vi "wd_repalceInIndex (DBL).vi"(6 "data type":T7, 7 "data":dbl[](array[numeric]), 8 "error in (no error)":errorcluster, 9 "value index":u64, 10 "channel index":u32, 11 "meta in":T1={"TargetFile"=path "", "StreamMode"=enum."File", "Append?"=FALSE, "ChunkSize"=0, "TimeColumnMode"=enum."Empty", "TimestampFormat"="", "AbsoluteTime?"=FALSE, "FileAttribute "={"Creator"="", "Title"="", "SheetName"=""}, "Column"=[], "FileRef"=refnum, "MemoryRef"=[], "RecordInfo"=[], " ChannelPreviousInfo"=[], "ChannelFirstRecord"=[], "PredefinedFormattedValueLength"=20, "DiskTemplate"={"XMLRef"=[refnum, refnum, refnum, refnum, refnum, refnum], "ZipPath"=path "", "MetaFile"={"Ref"=refnum, "NextRow"=0, "NextPosition"=0, "Block"=[]}, "TempFolder"=path ""}}) -> (0 "error out":errorcluster, 3 "meta out":T1={"TargetFile"=path "", "StreamMode"=enum."File", "Append?"=FALSE, "ChunkSize"=0, "TimeColumnMode"=enum."Empty", "TimestampFormat"="", "AbsoluteTime?"=FALSE, "FileAttribute "={"Creator"="", "Title"="", "SheetName"=""}, "Column"=[], "FileRef"=refnum, "MemoryRef"=[], "RecordInfo"=[], " ChannelPreviousInfo"=[], "ChannelFirstRecord"=[], "PredefinedFormattedValueLength"=20, "DiskTemplate"={"XMLRef"=[refnum, refnum, refnum, refnum, refnum, refnum], "ZipPath"=path "", "MetaFile"={"Ref"=refnum, "NextRow"=0, "NextPosition"=0, "Block"=[]}, "TempFolder"=path ""}})   [LabVIEW 2020, in "NI_ExcelFile.lvlib"]
uses:
  <vilib>/express/express shared/NI_ExcelFile/NI_ExcelFile.lvlib
  <vilib>/express/express shared/NI_ExcelFile/Ctrls/DataType.ctl
  <vilib>/express/express shared/NI_ExcelFile/Ctrls/MainData.ctl
  <vilib>/express/express shared/NI_ExcelFile/Ctrls/StreamMode.ctl
  <vilib>/express/express shared/NI_ExcelFile/Ctrls/TimeColumnMode.ctl
  <vilib>/express/express shared/NI_ExcelFile/Ctrls/FileAttribute.ctl
  <vilib>/express/express shared/NI_ExcelFile/Ctrls/Columns.ctl
  <vilib>/express/express shared/NI_ExcelFile/Ctrls/ColumnInfo.ctl
  <vilib>/express/express shared/NI_ExcelFile/Ctrls/wd_recordInfo.ctl
  <vilib>/express/express shared/NI_ExcelFile/Ctrls/disk_TemplateFile.ctl
  <vilib>/express/express shared/NI_ExcelFile/Ctrls/meta_file.ctl
  <vilib>/express/express shared/NI_ExcelFile/Ctrls/meta_Block.ctl
  <vilib>/express/express shared/NI_ExcelFile/Ctrls/meta_BlockType.ctl
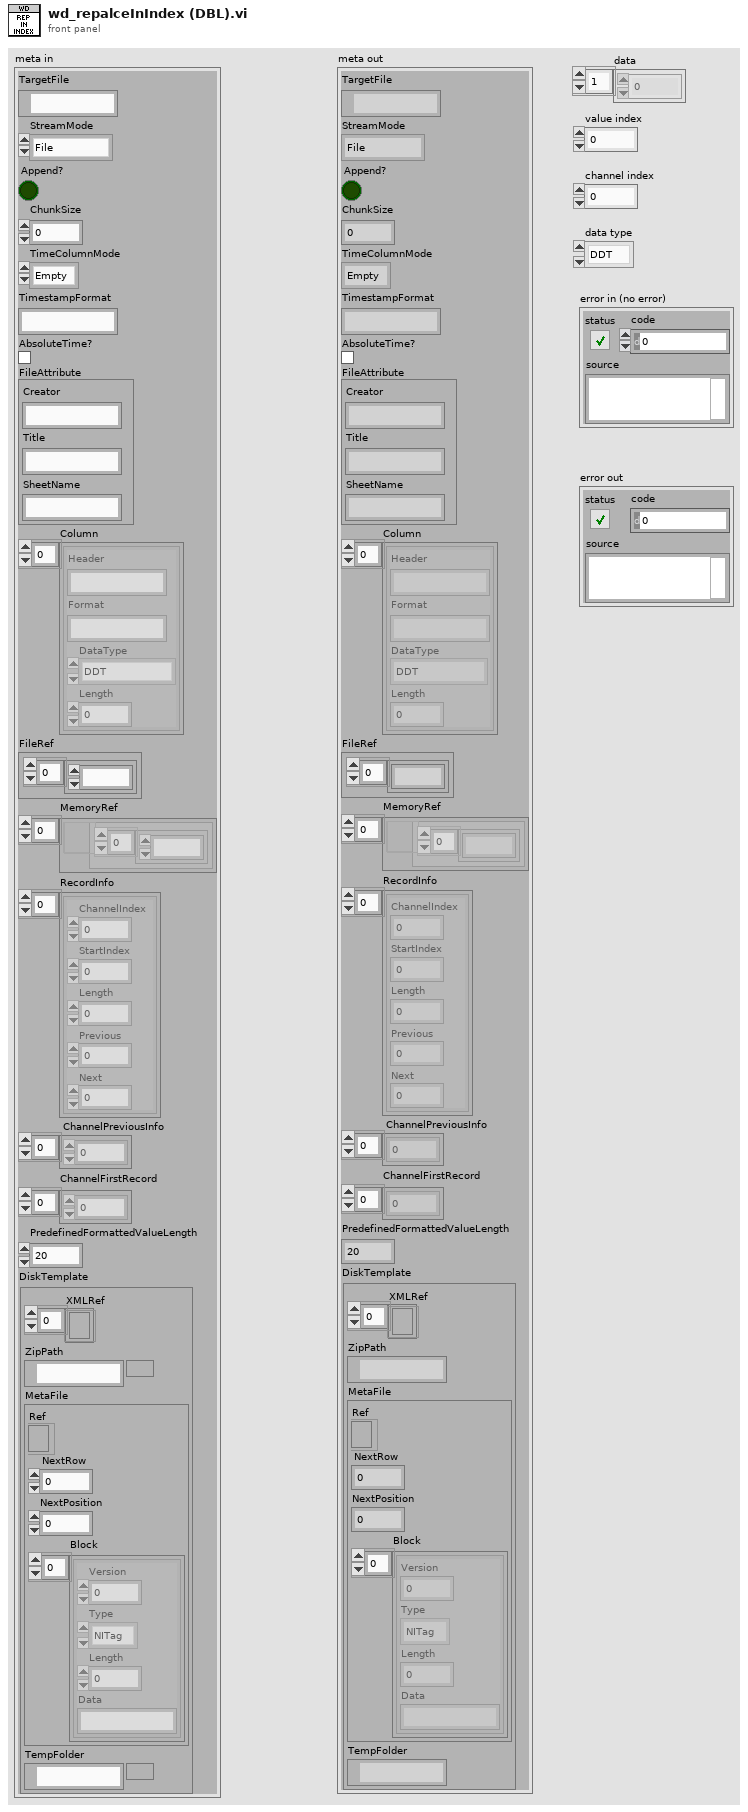
[diagram p1: front panel]
types:
  T1 = typedef "NI_ExcelFile.lvlib/MainData.ctl" = cluster{"TargetFile":path, "StreamMode":T2, "Append?":bool, "ChunkSize":u64, "TimeColumnMode":T3, "TimestampFormat":string, "AbsoluteTime?":bool, "FileAttribute ":T4, "Column":T5, "FileRef":refnum<k1>, "MemoryRef":refnum<data-value>[], "RecordInfo":T8[], " ChannelPreviousInfo":u32[], "ChannelFirstRecord":u32[], "PredefinedFormattedValueLength":i64, "DiskTemplate":T9}
  T2 = typedef "NI_ExcelFile.lvlib/StreamMode.ctl" = enum16{"File", "Memory"}
  T3 = typedef "NI_ExcelFile.lvlib/TimeColumnMode.ctl" = enum16{"Empty", "OnePerCh", "One"}
  T4 = typedef "NI_ExcelFile.lvlib/FileAttribute.ctl" = cluster{"Creator":string, "Title":string, "SheetName":string}
  T5 = typedef "NI_ExcelFile.lvlib/Columns.ctl" = T6[]
  T6 = typedef "NI_ExcelFile.lvlib/ColumnInfo.ctl" = cluster{"Header":string, "Format":string, "DataType":T7, "Length":u64}
  T7 = typedef "NI_ExcelFile.lvlib/DataType.ctl" = enum16{"DDT", "WFM", "Array of STR", "Array of DBL", "Array of I8", "Array of I16", "Array of I32", "Array of I64", "Array of SGL", "Array of U8", "Array of U16", "Array of U32", "Array of U64", "Array of Time"}
  T8 = typedef "NI_ExcelFile.lvlib/wd_recordInfo.ctl" = cluster{"ChannelIndex":u32, "StartIndex":u64, "Length":u64, "Previous":i32, "Next":i32}
  T9 = typedef "NI_ExcelFile.lvlib/disk_TemplateFile.ctl" = cluster{"XMLRef":refnum<file>[], "ZipPath":path, "MetaFile":T10, "TempFolder":path}
  T10 = typedef "NI_ExcelFile.lvlib/meta_file.ctl" = cluster{"Ref":refnum<file>, "NextRow":i32, "NextPosition":i64, "Block":T11[]}
  T11 = typedef "NI_ExcelFile.lvlib/meta_Block.ctl" = cluster{"Version":u16, "Type":T12, "Length":i32, "Data":string}
  T12 = typedef "NI_ExcelFile.lvlib/meta_BlockType.ctl" = enum16{"NITag", "File", "Column"}
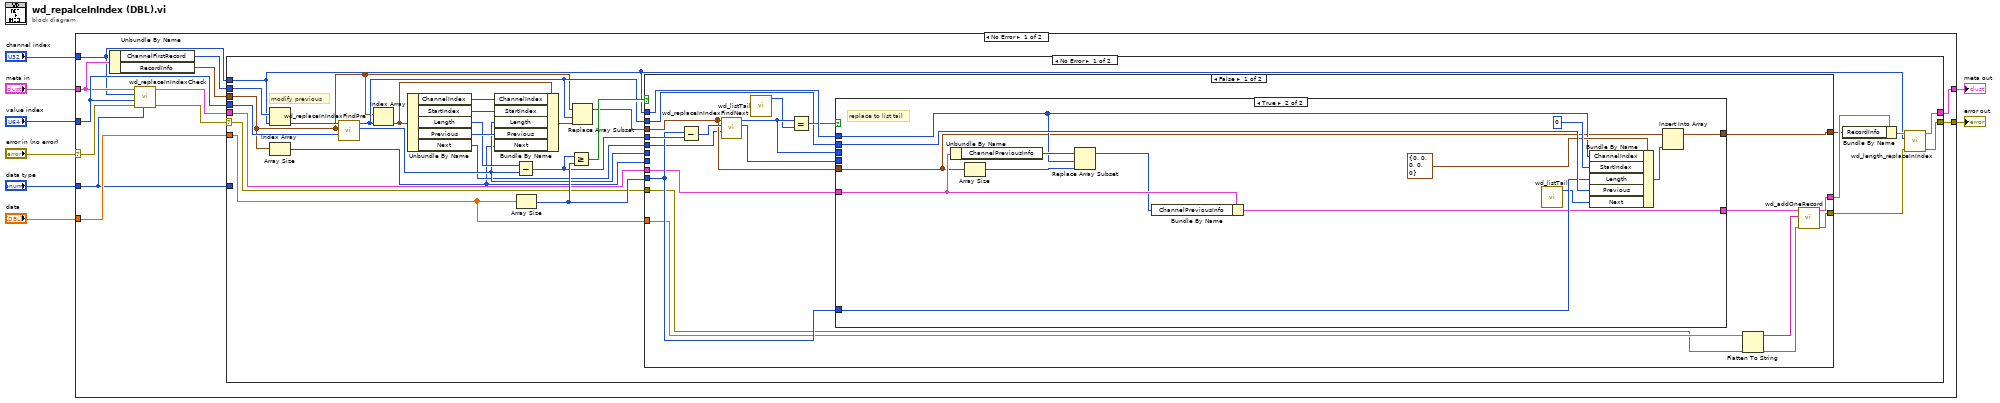
[diagram p0: block diagram]
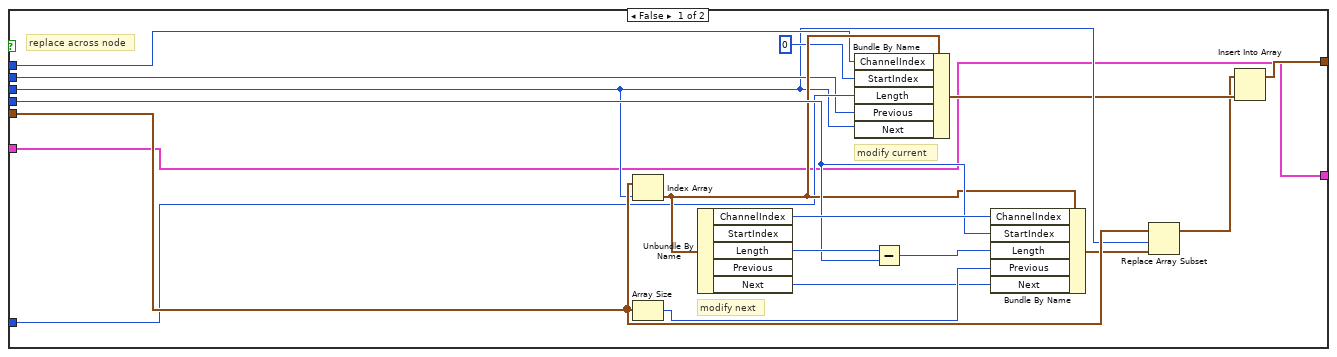
[diagram p2: hidden frame]
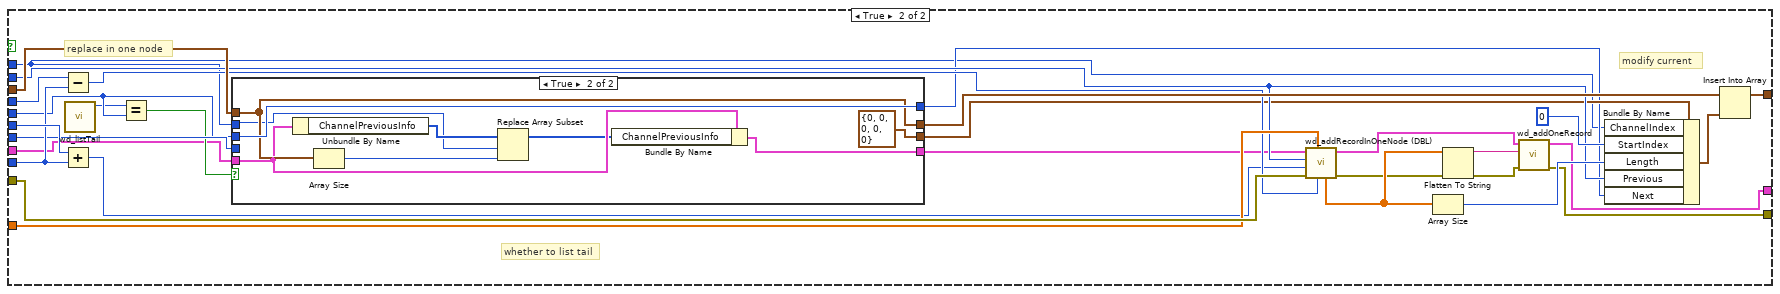
[diagram p3: hidden frame]
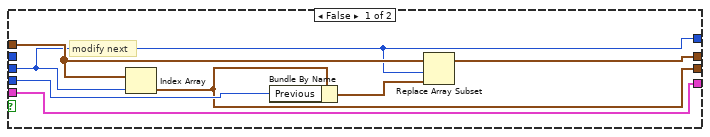
[diagram p4: hidden frame]
diagram:
  n1 = case shown="No Error" "error in (no error)" {
    selector: "error in (no error)" -> [w10 w150]
    tunnel: "channel index" -> [w13 _]
    tunnel: "meta in" -> [w14 w149]
    tunnel: "value index" -> [w17 _]
    tunnel: [w20 w150] -> w5
    tunnel: [w19 w149] -> w4
    tunnel: "data" -> [w18 _]
    tunnel: "data type" -> [w11 _]
    frame No Error {
      n2 = Unbundle By Name(w14) -> ("ChannelFirstRecord"=w16:u32[], "RecordInfo"=w15:T8[])
      n3 = call <vilib>:"wd_replaceInIndexCheck.vi"("data type"=w11, "error in (no error)"=w10, "value index"=w17, "channel index"=w13, "meta in"=w14) -> ("error out"=w9:errorcluster, "meta out"=w12:T1)  [unwired: 5 in]
      n4 = case shown="No Error" w9 {
        selector: w9 -> [w23 w147]
        tunnel: w12 -> [w33 w148]
        tunnel: w18 -> [w32 _]
        tunnel: [w28 w148] -> w19
        tunnel: [w21 w147] -> w20
        tunnel: w13 -> [w24 _]
        tunnel: w17 -> [w47 _]
        tunnel: w16 -> [w30 _]
        tunnel: w15 -> [w29 _]
        tunnel: w11 -> [_ _]
        frame No Error {
          # "modify previous"
          n5 = Index Array(array=w30, index=w24) -> (element=w48:u32)
          n6 = Array Size(array=w29) -> (size(s)=w34:i32)
          n7 = call <vilib>:"wd_replaceInIndexFindPre.vi"("value index"=w47, "RecordInfo"=w29, "node start index"=w48) -> ("value index out"=w38:u64, "pre node index"=w39:i32)  [unwired: 7 in]
          n8 = Index Array(array=w29, index=w39) -> (element=w31:T8)
          n9 = Unbundle By Name(w31) -> ("ChannelIndex"=w46:u32, "StartIndex"=w45:u64, "Length"=w42:u64, "Previous"=w44:i32, "Next"=w36:i32)
          n10 = Bundle By Name(cluster=w31, "ChannelIndex"=w46, "StartIndex"=w45, "Length"=w38, "Previous"=w44, "Next"=w34) -> (w43:T8)
          n11 = Subtract(x=w42, y=w38) -> (x-y=w37:u64)
          n12 = Array Size(array=w32) -> (size(s)=w40:i32)
          n13 = Greater Or Equal?(x=w37, y=w40) -> (x >= y?=w41:bool)
          n14 = Replace Array Subset(array=w29, new element=w43, index=w39) -> (w35:T8[])
          n15 = case shown="False" w41 {
            tunnel: w24 -> [w64 w102]
            tunnel: w40 -> [w65 w127]
            tunnel: w39 -> [w51 w113]
            tunnel: w33 -> [w58 w104]
            tunnel: w32 -> [w55 w117]
            tunnel: w38 -> [_ w129]
            tunnel: w37 -> [w68 w128]
            tunnel: w36 -> [w50 w107]
            tunnel: w35 -> [w61 w122]
            tunnel: [w66 w123] -> w25
            tunnel: w34 -> [_ w126]
            tunnel: [w56 w118] -> w27
            tunnel: w23 -> [w53 w120]
            tunnel: [w59 w119] -> w22
            frame False {
              n16 = Subtract(x=w65, y=w68) -> (x-y=w67:u64)
              n17 = call <vilib>:"wd_replaceInIndexFindNext.vi"("Next in"=w50, "LengthIn"=w67, "RecordInfo"=w61) -> ("LengthOut"=w62:u64, "Next out"=w60:i32)  [unwired: 7 in]
              n18 = call <vilib>:"wd_listTail.vi"() -> ("list tail"=w49:i32)  [unwired: 11 in]
              n19 = Equal?(x=w60, y=w49) -> (x = y?=w63:bool)
              n20 = case shown="True" w63 {
                tunnel: w61 -> [w80 w88]
                tunnel: w60 -> [w73 _]
                tunnel: w62 -> [w83 _]
                tunnel: [w70 w90] -> w66
                tunnel: w64 -> [w77 w89]
                tunnel: w65 -> [w75 w96]
                tunnel: w51 -> [w74 w99]
                tunnel: w58 -> [w69 w94]
                tunnel: [w69 w92] -> w57
                frame False {
                  # "replace across node"
                  # "modify current"
                  # "modify next"
                  n21 = Index Array(array=w80, index=w73) -> (element=w78:T8)
                  n22 = Array Size(array=w80) -> (size(s)=w82:i32)
                  n23 = Unbundle By Name(w78) -> ("ChannelIndex"=w86:u32, "Length"=w84:u64, "Next"=w81:i32)  [unwired: 2 out]
                  n24 = Bundle By Name(cluster=w78, "ChannelIndex"=w77, "StartIndex"=u64 0 ("Start Index"), "Length"=w75, "Previous"=w74, "Next"=w73) -> (w72:T8)
                  n25 = Subtract(x=w84, y=w83) -> (x-y=w85:u64)
                  n26 = Bundle By Name(cluster=w78, "ChannelIndex"=w86, "StartIndex"=w83, "Length"=w85, "Previous"=w82, "Next"=w81) -> (w79:T8)
                  n27 = Replace Array Subset(array=w80, new element=w79, index=w73) -> (w71:T8[])
                  n28 = Insert Into Array(array=w71, new element=w72) -> (w70:T8[])  [unwired: 1 in]
                }
                frame True {
                  # "replace to list tail"
                  n29 = Unbundle By Name(w94) -> ("ChannelPreviousInfo"=w97:u32[])
                  n30 = Array Size(array=w88) -> (size(s)=w95:i32)
                  n31 = Replace Array Subset(array=w97, new element=w95, index=w89) -> (w93:u32[])
                  n32 = Bundle By Name(cluster=w94, "ChannelPreviousInfo"=w93) -> (w92:T1)
                  n33 = call <vilib>:"wd_listTail.vi"() -> ("list tail"=w87:i32)  [unwired: 11 in]
                  n34 = Bundle By Name(cluster=T8 {"ChannelIndex"=0, "StartIndex"=0, "Length"=0, "Previous"=0, "Next"=0} ("output cluster"), "ChannelIndex"=w89, "StartIndex"=u64 0 ("Start Index"), "Length"=w96, "Previous"=w99, "Next"=w87) -> (w98:T8)
                  n35 = Insert Into Array(array=w88, new element=w98) -> (w90:T8[])  [unwired: 1 in]
                }
              }
              n36 = Flatten To String(anything=w55, error in (no error)=w53) -> (data string=w54:string, error out=w52:errorcluster)  [unwired: 2 in, 1 out]
              n37 = call <vilib>:"wd_addOneRecord.vi"("error in (no error)"=w52, "data"=w54, "meta in"=w57) -> ("error out"=w59:errorcluster, "meta out"=w56:T1)  [unwired: 7 in]
            }
            frame True {
              # "whether to list tail"
              # "replace in one node"
              # "modify current"
              n38 = Subtract(x=w128, y=w127) -> (x-y=w115:u64)
              n39 = Add(x=w129, y=w127) -> (x+y=w114:u64)
              n40 = call <vilib>:"wd_listTail.vi"() -> ("list tail"=w101:i32)  [unwired: 11 in]
              n41 = Equal?(x=w101, y=w107) -> (x = y?=w106:bool)
              n42 = case shown="True" w106 {
                tunnel: w126 -> [w137 _]
                tunnel: [w135 w144] -> w125
                tunnel: w122 -> [w134 w144]
                tunnel: [w133 T8 {"ChannelIndex"=0, "StartIndex"=0, "Length"=0, "Previous"=0, "Next"=0} ("RecordInfo")] -> w112
                tunnel: w107 -> [w132 w145]
                tunnel: [w132 w145] -> w105
                tunnel: w104 -> [w131 w140]
                tunnel: [w131 w138] -> w103
                tunnel: w102 -> [_ w142]
                frame False {
                  # "modify next"
                  n43 = Index Array(array=w134, index=w132) -> (element=w133:T8)
                  n44 = Bundle By Name(cluster=w133, "Previous"=w137) -> (w136:T8)
                  n45 = Replace Array Subset(array=w134, new element=w136, index=w132) -> (w135:T8[])
                }
                frame True {
                  n46 = Unbundle By Name(w140) -> ("ChannelPreviousInfo"=w143:u32[])
                  n47 = Array Size(array=w144) -> (size(s)=w141:i32)
                  n48 = Replace Array Subset(array=w143, new element=w141, index=w142) -> (w139:u32[])
                  n49 = Bundle By Name(cluster=w140, "ChannelPreviousInfo"=w139) -> (w138:T1)
                }
              }
              n50 = call <vilib>:"wd_addRecordInOneNode (DBL).vi"("length"=w115, "data"=w117, "error in (no error)"=w120, "start"=w114, "datalog postion"=w113, "meta in"=w103) -> ("error out"=w109:errorcluster, "meta out"=w116:T1, "data subset"=w111:dbl[])  [unwired: 3 in]
              n51 = Array Size(array=w111) -> (size(s)=w121:i32)
              n52 = Flatten To String(anything=w111, error in (no error)=w109) -> (data string=w110:string, error out=w108:errorcluster)  [unwired: 2 in, 1 out]
              n53 = call <vilib>:"wd_addOneRecord.vi"("error in (no error)"=w108, "data"=w110, "meta in"=w116) -> ("error out"=w119:errorcluster, "meta out"=w118:T1)  [unwired: 7 in]
              n54 = Bundle By Name(cluster=w112, "ChannelIndex"=w102, "StartIndex"=u64 0 ("Start Index"), "Length"=w121, "Previous"=w113, "Next"=w105) -> (w124:T8)
              n55 = Insert Into Array(array=w125, new element=w124) -> (w123:T8[])  [unwired: 1 in]
            }
          }
          n56 = Bundle By Name(cluster=w27, "RecordInfo"=w25) -> (w26:T1)
          n57 = call <vilib>:"wd_length_replaceInIndex.vi"("error in (no error)"=w22, "channel index"=w24, "meta in"=w26) -> ("error out"=w21:errorcluster, "meta out"=w28:T1)  [unwired: 7 in]
        }
        frame Error {
        }
      }
    }
    frame Error {
    }
  }
  "error out" <- w5
  "meta out" <- w4
